vi "(main) Stablize z-axis.vi"() -> ()   [LabVIEW 2014]
uses:
  Main-Stage-PI/(Global) Current handle and LaserPower_YCC.vi
  Global 1 extract image.vi
  <vilib>/Analysis/polynomials.llb/Scalar Polynomial Evaluation (DBL).vi
  <vilib>/Utility/file.llb/Write To Spreadsheet File (DBL).vi
  <vilib>/Analysis/NI_AALPro.lvlib
panel:
  in  "manual set?":bool
  in  "manual set amp.":dbl
  in  "scan cycle":i32=1
  out "set amp.":dbl
  out "current amp.":dbl
  in  "PID gains":T1={"proportional gain (Kc)"=0.0089999, "integral time (Ti, min)"=0.5000001, "derivative time (Td, min)"=0.0} {"derivative time (Td, min)" format="%.8f"; "integral time (Ti, min)" format="%.8f"; "proportional gain (Kc)" format="%.8f"}
  in  "ms to wait for PID":u32=50
  in  "PID output range":cluster{"output high":dbl, "output low":dbl}={"output high"=51.0, "output low"=49.0} {"output low" format="%.2f"; "output high" format="%.2f"}
  in  "stop PID feedback":bool
  in  "save feedback data?":bool
  in  "save calib. curve?":bool
  in  "T=feedback; F=not":bool=TRUE
  out "Z position":dbl
  in  "set height (nm)":dbl
  out "upper":dbl
  out "lower":dbl
  in  "1/2 scan range (um)":dbl=0.30000000000000004
  in  "step number":i32=30
  in  "Select Ref. \npeak location":dbl=7.0
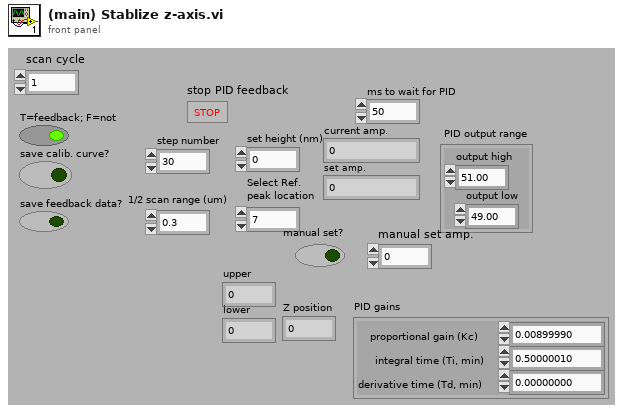
[diagram p1: front panel]
types:
  T1 = cluster{"proportional gain (Kc)":dbl, "integral time (Ti, min)":dbl, "derivative time (Td, min)":dbl}
  T2 = typedef "IMAQ Image.ctl" = refnum<image>
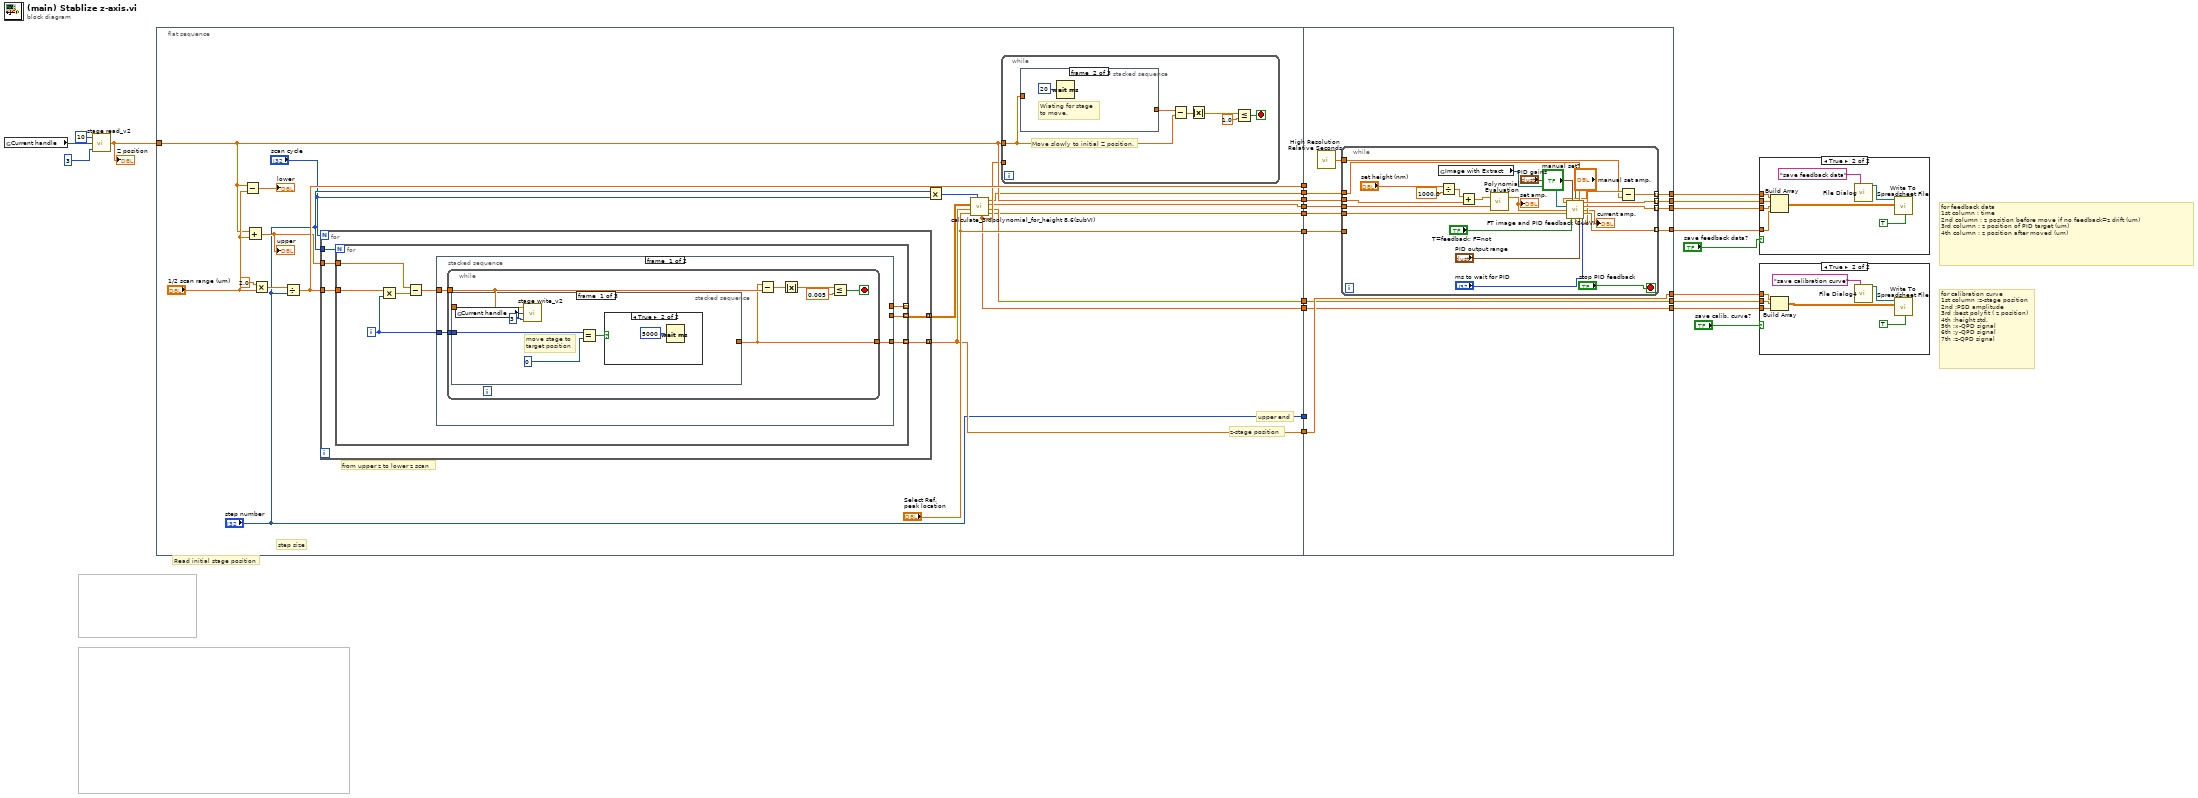
[diagram p0: block diagram]
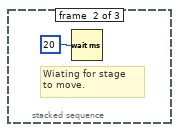
[diagram p5: hidden frame]
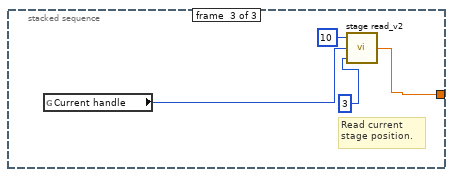
[diagram p6: hidden frame]
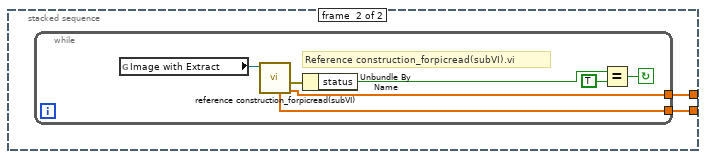
[diagram p7: hidden frame]
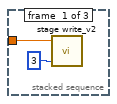
[diagram p8: hidden frame]
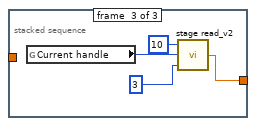
[diagram p9: hidden frame]
diagram:
  # "for feedback data\n1st column : time\n2nd column : z position before move if no feedback=z drift (um) \n3rd column : z position of PID target (um)\n4th column : z position after moved (um)"
  # "for calibration curve\n1st column :z-stage position\n2nd :PSD amplitude\n3rd :best polyfit ( z position) \n4th :height std.\n5th :x-QPD signal\n6th :y-QPD signal\n7th :z-QPD signal"
  # "Read initial stage position"
  n1 = global read "(Global) Current handle and LaserPower_YCC.vi" "Current handle"() -> (w2:i32)
  n2 = call "stage read_v2.vi"("Axis"=u32 3 ("axis"), "Incoming Handle"=w2, "read #"=10) -> ("position (um)"=w3:dbl)  [unwired: 1 in, 1 out]
  "Z position" <- w3
  n3 = flat-sequence {
    tunnel: w3 -> [w34]
    tunnel: ["step number"] -> w23
    tunnel: [w38] -> w22
    tunnel: ["Select Ref. \npeak location"] -> w21
    tunnel: [w34] -> w20
    tunnel: [w32] -> w17
    tunnel: [w33] -> w15
    tunnel: [w31] -> w10
    tunnel: [w30] -> w9
    tunnel: [w29] -> w6
    tunnel: [w24] -> w5
    tunnel: w23 -> [_]
    tunnel: w22 -> [_]
    tunnel: w21 -> [w111]
    tunnel: w20 -> [w110]
    tunnel: [w109] -> w18
    tunnel: w17 -> [w109]
    tunnel: [w108] -> w16
    tunnel: w15 -> [w108]
    tunnel: [w103] -> w13
    tunnel: [w107] -> w12
    tunnel: [w106] -> w11
    tunnel: w10 -> [w105]
    tunnel: w9 -> [w104]
    tunnel: [w101] -> w8
    tunnel: [w100] -> w7
    tunnel: w6 -> [w100]
    tunnel: w5 -> [w99]
    frame #0 {
      # "z-stage position"
      # "from upper z to lower z scan"
      # "upper end"
      # "step size"
      n4 = Subtract(x=w34, y="1/2 scan range (um)") -> (x-y=→"lower":dbl)
      n5 = Add(x=w34, y="1/2 scan range (um)") -> (x+y=w36:dbl)
      "upper" <- w36
      n6 = Multiply(x=2.0, y="1/2 scan range (um)") -> (x*y=w39:dbl)
      n7 = Divide(x=w39, y="step number") -> (x/y=w38:dbl)
      n8 = for {
        N: "scan cycle" -> [_]
        tunnel: w38 -> [w46]
        tunnel: "step number" -> [w45]
        tunnel: w36 -> [w44]
        tunnel: [w43] -> w32 mode=concatenating
        tunnel: [w42] -> w28 mode=concatenating
        n9 = for {
          N: w45 -> [_]
          tunnel: w46 -> [w54]
          tunnel: w44 -> [w51]
          tunnel: [w50] -> w43 mode=indexing
          tunnel: [w48] -> _ mode=indexing
          tunnel: [w47] -> w42 mode=indexing
          i -> [w49]
          n10 = Multiply(x=w54, y=w49) -> (x*y=w53:dbl)
          n11 = Subtract(x=w51, y=w53) -> (x-y=w52:dbl)
          n12 = stacked-sequence {
            tunnel: [w56 _] -> w50
            tunnel: w52 -> [w57 _]
            tunnel: w49 -> [w55 _]
            tunnel: [_ w78] -> w48
            tunnel: [_ w77] -> w47
            frame #0 {
              n13 = while {
                tunnel: w57 -> [w64]
                tunnel: [w59] -> w56
                tunnel: w55 -> [w58]
                stop <- w60 stop-if-true
                n14 = stacked-sequence {
                  tunnel: w64 -> [w67 _ _]
                  tunnel: [_ _ w76] -> w59
                  tunnel: w58 -> [w68 _ _]
                  frame #0 {
                    # "move stage to \ntarget position"
                    n15 = global read "(Global) Current handle and LaserPower_YCC.vi" "Current handle"() -> (w65:i32)
                    n16 = call "stage write_v2.vi"("axis"=u32 3, "Incoming Handle"=w65, "position"=w67) -> ()  [unwired: 2 in, 1 out]
                    n17 = Equal?(x=w68, y=0) -> (x = y?=w70:bool)
                    n18 = case shown="True" w70 {
                      frame False {
                      }
                      frame True {
                        n19 = Wait (ms)(milliseconds to wait=u32 5000) -> ()  [unwired: 1 out]
                      }
                    }
                  }
                  frame #1 {
                    # "Wiating for stage \nto move."
                    n20 = Wait (ms)(milliseconds to wait=u32 20) -> ()  [unwired: 1 out]
                  }
                  frame #2 {
                    # "Read current \nstage position."
                    n21 = global read "(Global) Current handle and LaserPower_YCC.vi" "Current handle"() -> (w74:i32)
                    n22 = call "stage read_v2.vi"("Axis"=u32 3 ("axis"), "Incoming Handle"=w74, "read #"=10) -> ("position (um)"=w76:dbl)  [unwired: 1 in, 1 out]
                  }
                }
                n23 = Subtract(x=w59, y=w64) -> (x-y=w63:dbl)
                n24 = Absolute Value(x=w63) -> (abs(x)=w62:dbl)
                n25 = Less Or Equal?(x=w62, y=0.005) -> (x <= y?=w60:bool)
              }
            }
            frame #1 {
              n26 = while {
                tunnel: [w82] -> w78
                tunnel: [w81] -> w77
                stop <- w83 continue-if-true
                # "Reference construction_forpicread(subVI).vi"
                n27 = global read "Global 1 extract image.vi" "Image with Extract"() -> (w85:T2)
                n28 = call "reference construction_forpicread(subVI).vi"("Image in"=w85) -> ("Waveform Graph 2"=w82:dbl[], "error out"=w80:errorcluster, "Power Spectrum"=w81:dbl[])  [unwired: 6 in, 2 out]
                n29 = Unbundle By Name(w80) -> ("status"=w79:bool)
                n30 = Equal?(x=w79, y=TRUE) -> (x = y?=w83:bool)
              }
            }
          }
        }
      }
      n31 = Multiply(x="step number", y="scan cycle") -> (x*y=w25:i32)
      n32 = call "calculate_3rdpolynomial_for_height 8.6(subVI).vi"("Total pic. #"=w25, "Selected \nPeak Location"="Select Ref. \npeak location", "Z axis height"=w32, "Amplitude"=w28) -> ("Selected \nPeak Location out"=w24:dbl, "cali-amp."=w29:dbl[], "Polynomial Coefficients\n(position to amp.)"=w31:dbl[], "Polynomial Coefficients\n(amp. to position)"=w30:dbl[], "Best Polynomial Fit"=w33:dbl[])  [unwired: 2 in, 1 out]
      n33 = while {
        tunnel: w34 -> [w87]
        tunnel: w33 -> [_]
        stop <- w88 stop-if-true
        # "Move slowly to initial Z position."
        n34 = stacked-sequence {
          tunnel: w87 -> [w93 _ _]
          tunnel: [_ _ w95] -> w86
          frame #0 {
            n35 = call "stage write_v2.vi"("axis"=u32 3, "position"=w93) -> ()  [unwired: 3 in, 1 out]
          }
          frame #1 {
            # "Wiating for stage \nto move."
            n36 = Wait (ms)(milliseconds to wait=u32 20) -> ()  [unwired: 1 out]
          }
          frame #2 {
            n37 = global read "(Global) Current handle and LaserPower_YCC.vi" "Current handle"() -> (w97:i32)
            n38 = call "stage read_v2.vi"("Axis"=u32 3 ("axis"), "Incoming Handle"=w97, "read #"=10) -> ("position (um)"=w95:dbl)  [unwired: 1 in, 1 out]
          }
        }
        n39 = Subtract(x=w86, y=w87) -> (x-y=w91:dbl)
        n40 = Absolute Value(x=w91) -> (abs(x)=w90:dbl)
        n41 = Less Or Equal?(x=w90, y=1.0) -> (x <= y?=w88:bool)
      }
    }
    frame #1 {
      n42 = call <vilib>:"High Resolution Relative Seconds.vi"() -> ("relative seconds"=w102:dbl)
      n43 = while {
        tunnel: w111 -> [_]
        tunnel: w110 -> [w130]
        tunnel: [w128] -> w107 mode=indexing
        tunnel: [w127] -> w106 mode=indexing
        tunnel: w105 -> [w117]
        tunnel: w104 -> [w126]
        tunnel: [w129] -> w103 mode=indexing
        tunnel: w102 -> [w121]
        tunnel: [w120] -> w101 mode=indexing
        tunnel: w99 -> [w116]
        stop <- "stop PID feedback" stop-if-true
        n44 = global read "Global 1 extract image.vi" "Image with Extract"() -> (w135:T2)
        n45 = Divide(x="set height (nm)", y=1000.0) -> (x/y=w131:dbl)
        n46 = Add(x=w131, y=w130) -> (x+y=w115:dbl)
        n47 = call-poly <vilib>:"Polynomial Evaluation.vi"("P(x)"=w117, "a"=w115) -> ("P(a)"=w114:dbl)  [unwired: 1 out]
        "set amp." <- w114
        n48 = call "FT image and PID feedback (SubVI).vi"("manual set amp."="manual set amp.", "PID gains"="PID gains", "manual set?"="manual set?", "Polyfit Coeff. \n(amp. to position)"=w126, "Image with Extract"=w135, "set amp."=w114, "select fre."=w116, "T=feedback; F=not"="T=feedback; F=not", "output range"="PID output range", "ms to wait for PID"="ms to wait for PID") -> ("z position before move\nor no feedback=z drift (um)"=w128:dbl, "z position of PID target (um)"=w129:dbl, "current amp."=→"current amp.":dbl, "z position after moved (um)"=w127:dbl, "relative seconds"=w122:dbl)  [unwired: 1 in]
        n49 = Subtract(x=w122, y=w121) -> (x-y=w120:dbl)
      }
    }
  }
  n50 = case shown="True" "save feedback data?" {
    tunnel: w13 -> [_ w141]
    tunnel: w12 -> [_ w140]
    tunnel: w11 -> [_ w139]
    tunnel: w8 -> [_ w136]
    frame False {
    }
    frame True {
      n51 = Build Array(w136, w140, w141, w139) -> (w137:dbl[][])
      n52 = call "File Dialog"("prompt"="save feedback data") -> ("selected path"=w143:path)  [unwired: 11 in, 3 out]
      n53 = call-poly <vilib>:"Write To Spreadsheet File.vi"("transpose? (no:F)"=TRUE, "2D data"=w137, "file path (dialog if empty)"=w143) -> ()  [unwired: 3 in, 3 out]
    }
  }
  n54 = case shown="True" "save calib. curve?" {
    tunnel: w18 -> [_ w149]
    tunnel: w16 -> [_ w145]
    tunnel: w7 -> [_ w144]
    frame False {
    }
    frame True {
      n55 = Build Array(w149, w144, w145) -> (w150:dbl[][])
      n56 = call "File Dialog4"("prompt"="save calibration curve") -> ("selected path"=w147:path)  [unwired: 11 in, 3 out]
      n57 = call-poly <vilib>:"Write To Spreadsheet File.vi"("transpose? (no:F)"=TRUE, "2D data"=w150, "file path (dialog if empty)"=w147) -> ()  [unwired: 3 in, 3 out]
    }
  }
